vi "readXML.vi"(8 "error in (no error)":errorcluster, 10 "Path":path, 11 "WinX32Settings in":refnum<class "WinX32Settings.lvclass">) -> (0 "error out":errorcluster, 3 "WinX32Settings out":refnum<class "WinX32Settings.lvclass">)   [LabVIEW 2011, in "Tools.lvlib" / "Settings.lvlib" / "WinX32Settings.lvclass"]
uses:
  WinX32Settings.lvclass
  NativeXML/NativeXML.lvclass
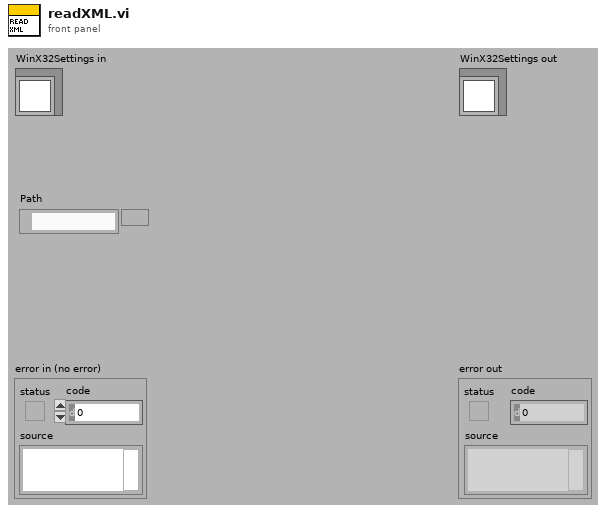
[diagram p1: front panel]
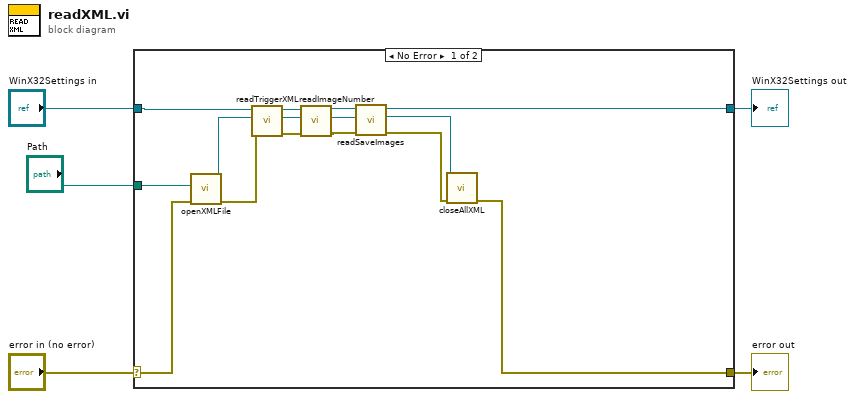
[diagram p0: block diagram]
diagram:
  n1 = case shown="No Error" "error in (no error)" {
    selector: "error in (no error)" -> [w20 w22]
    tunnel: [w6 w22] -> w4
    tunnel: [w7 w21] -> w2
    tunnel: "WinX32Settings in" -> [w18 w21]
    tunnel: "Path" -> [w19 _]
    frame No Error {
      n2 = call "openXMLFile.vi"("error in (no error)"=w20, "Path"=w19) -> ("error out"=w16:errorcluster, "NativeXML out"=w17:refnum<class "NativeXML.lvclass">)  [unwired: 8 in]
      n3 = call "readTriggerXML.vi"("error in (no error)"=w16, "NativeXML in"=w17, "WinX32Settings in"=w18) -> ("error out"=w14:errorcluster, "NativeXML out"=w13:refnum<class "NativeXML.lvclass">, "WinX32Settings out"=w15:refnum<class "WinX32Settings.lvclass">)  [unwired: 6 in]
      n4 = call "readImageNumber.vi"("error in (no error)"=w14, "NativeXML in"=w13, "WinX32Settings in"=w15) -> ("error out"=w10:errorcluster, "NativeXML out"=w11:refnum<class "NativeXML.lvclass">, "WinX32Settings out"=w12:refnum<class "WinX32Settings.lvclass">)  [unwired: 6 in]
      n5 = call "readSaveImages.vi"("error in (no error)"=w10, "NativeXML in"=w11, "WinX32Settings in"=w12) -> ("error out"=w9:errorcluster, "NativeXML out"=w8:refnum<class "NativeXML.lvclass">, "WinX32Settings out"=w7:refnum<class "WinX32Settings.lvclass">)  [unwired: 6 in]
      n6 = call "closeAllXML.vi"("error in (no error)"=w9, "NativeXML in"=w8) -> ("error out"=w6:errorcluster)  [unwired: 9 in]
    }
    frame Error {
    }
  }
  "error out" <- w4
  "WinX32Settings out" <- w2
